vi "main_target.vi"() -> ()   [LabVIEW 2011]
uses:
  Ctrls/command.ctl
  controls.llb/RTFIFO operate.ctl
panel:
  in  "variable":T2 {"command" items=["NO_Action", "start", "pause", "resum", "stop", "config", "System_constant", "7", "DAQ_init", "DAQ_config", "DAQ_start", "DAQ_read", "DAQ_stop", "DAQ_contrl", "14", "15", "16", "17", "18", "19", "Zsf_open", "Zsf_close", "Wkf_control", "Pump_switch", "dcf_switch", "JRQ_switch"]}
  in  "error in":errorcluster
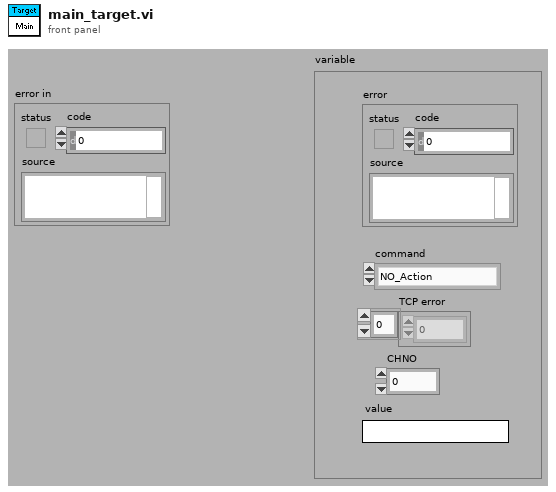
[diagram p1: front panel]
types:
  T1 = typedef "command.ctl" = u16
  T2 = cluster{"error":errorcluster, "TCP error":i32[], "command":T1, "CHNO":u16, "value":string}
  T3 = enum16{"connect", "receive data", "send data", "data transfer"}
  T4 = enum16{"connect", "receive data", "send data", "data transfer", "close"}
  T5 = typedef "RTFIFO operate.ctl" = enum16{"Creat", "Write", "Read", "Delete"}
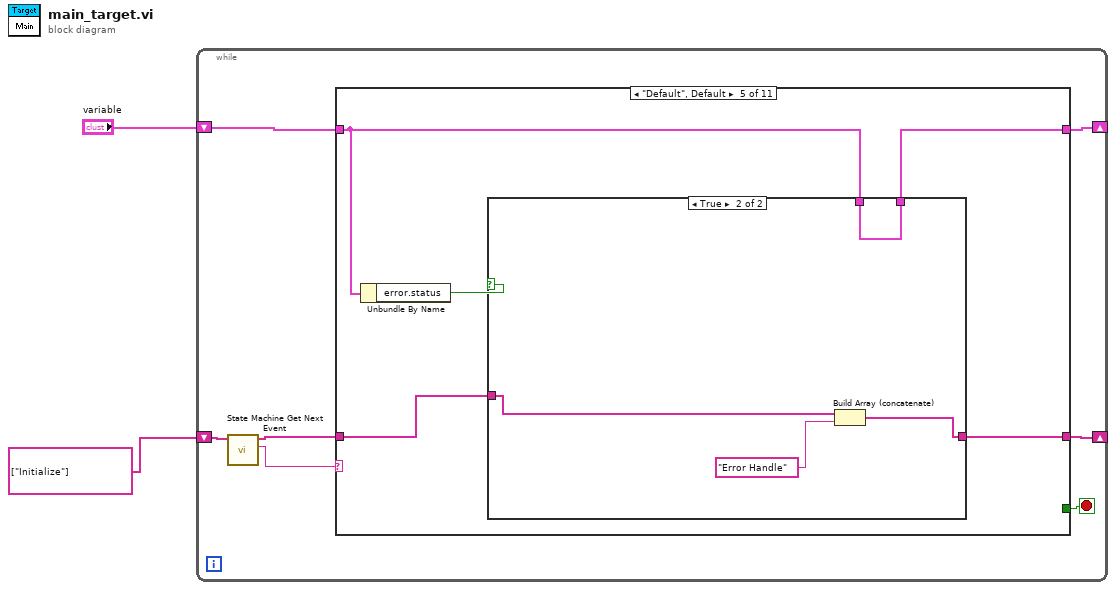
[diagram p0: block diagram]
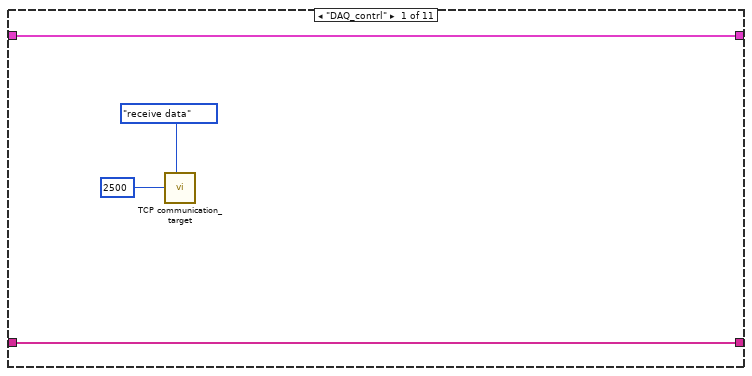
[diagram p2: hidden frame]
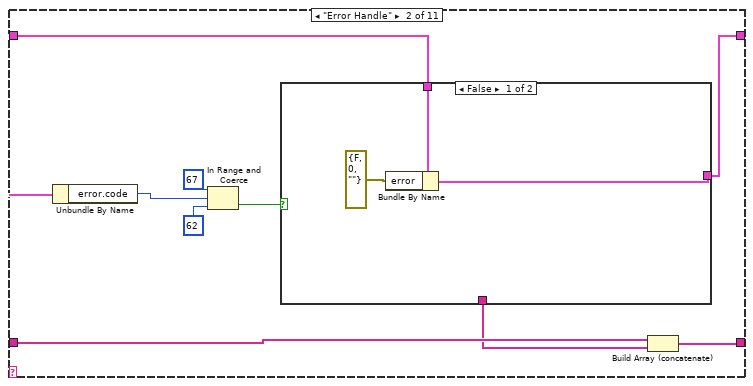
[diagram p3: hidden frame]
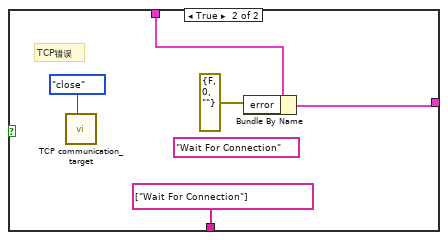
[diagram p4: hidden frame]
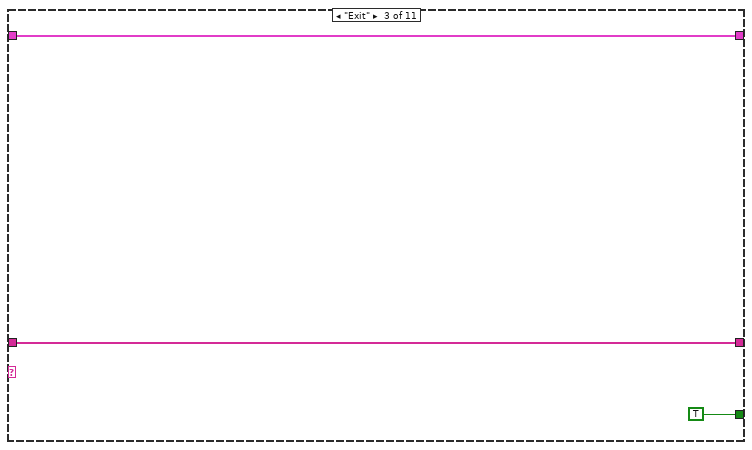
[diagram p5: hidden frame]
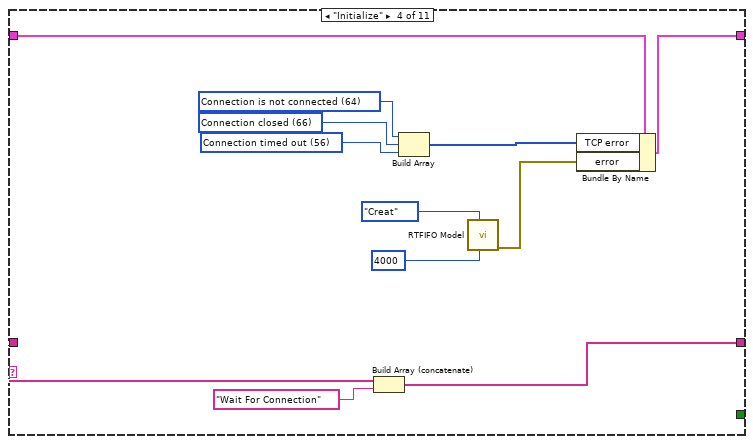
[diagram p6: hidden frame]
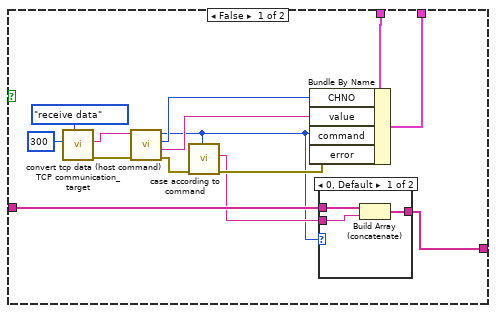
[diagram p7: hidden frame]
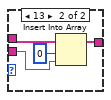
[diagram p8: hidden frame]
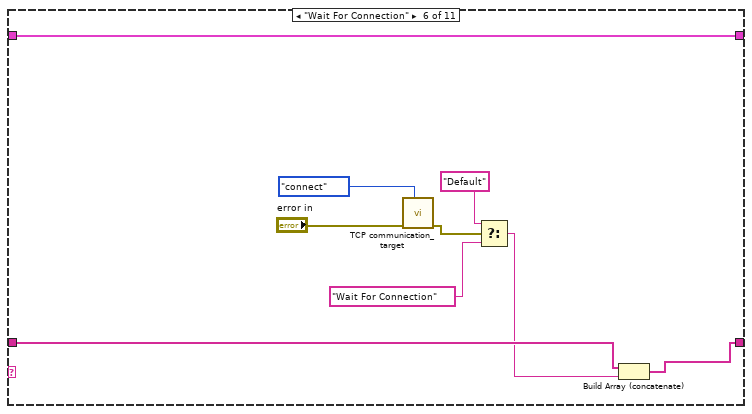
[diagram p9: hidden frame]
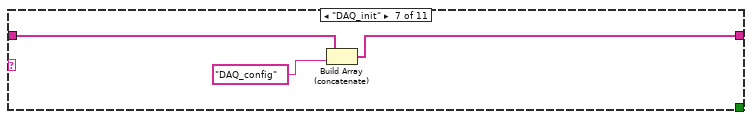
[diagram p10: hidden frame]
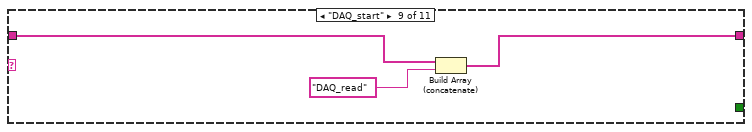
[diagram p12: hidden frame]
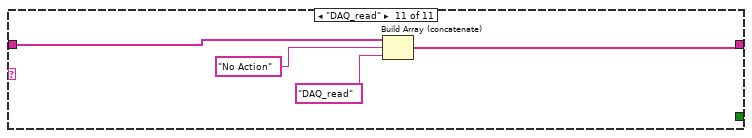
[diagram p14: hidden frame]
diagram:
  n1 = while {
    shift-right: [w5] -> _
    shift-left: string[] ["Initialize"] -> [w9]
    shift-right: [w3] -> _
    shift-left: "variable" -> [w4]
    stop <- w7 stop-if-true
    n2 = call "State Machine Get Next Event.vi"("event queue in"=w9) -> ("next event"=w8:string, "event queue out"=w6:string[])  [unwired: 5 in]
    n3 = case shown="\"Default\", Default" w8 {
      tunnel: [_ _ TRUE _ _ _ _ _ _ _ _] -> w7
      tunnel: w6 -> [w10 w20 w32 w45 w47 w78 w87 w88 w91 w93 w97]
      tunnel: [w10 w19 w32 w44 w46 w77 w86 w88 w89 w93 w96] -> w5
      tunnel: w4 -> [w13 w22 w31 w40 w50 w84 _ _ _ w92 _]
      tunnel: [w13 w21 w31 w39 w48 w84 _ _ _ w92 _] -> w3
      frame "DAQ_contrl" {
        n4 = call "TCP communication_target.vi"("TCP command"=T3."receive data", "timeout ms"=2500) -> ()  [unwired: 8 in, 2 out]
      }
      frame "Error Handle" {
        n5 = Unbundle By Name(w22) -> ("error.code"=w17:i32)
        n6 = In Range and Coerce(upper limit=67, x=w17, lower limit=62) -> (In Range?=w14:bool)  [unwired: 1 out]
        n7 = case shown="False" w14 {
          tunnel: w22 -> [w25 w29]
          tunnel: [w23 w28] -> w21
          tunnel: [_ string[] ["Wait For Connection"]] -> w18
          frame False {
            n8 = Bundle By Name(cluster=w25, "error"=errorcluster {"status"=FALSE, "code"=0, "source"=""}) -> (w23:T2)
          }
          frame True {
            (unwired) "Wait For Connection"
            # "TCP错误"
            n9 = call "TCP communication_target.vi"("TCP command"=T4."close") -> ()  [unwired: 9 in, 2 out]
            n10 = Bundle By Name(cluster=w29, "error"=errorcluster {"status"=FALSE, "code"=0, "source"=""}) -> (w28:T2)
          }
        }
        n11 = Build Array (concatenate)(w20, w18) -> (w19:string[])
      }
      frame "Exit" {
      }
      frame "Initialize" {
        w37 = 66 items=["No Error", "Argument Error", "Memory Full", "Out of Zone", "End of File", "File Already Open", "Generic File IO Error", "File Not Found", "File Permission Error", "Disk Full", "Duplicate Path", "Too Many Files Open", "Not Enabled", "Resource File Not Found", "Cannot Add Resource", "Resource Not Found", "Image Not Found", "Image Memory Error", "Pen Does Not Exist", "Config Bad Type", "Config Token Not Found", "Config Parse Error", "Config Memory Error", "Bad External Code Format", "Bad External Code Offset", "External Code Not Present", "Null Window", "Destroy Window Mixup", "Null Menu", "Print Aborted", "Bad Print Record", "Print Driver Error", "Windows Error During Print", "Memory Error During Print", "Print Dialog Error", "Generic Print Error", "Invalid Device Refnum", "Device Not Found", "Device Parameter Error", "Device Unit Error", "Can't Open Device", "Device Call Aborted", "Generic Error", "Cancelled By User", "Object ID Too Low", "Object ID Too High", "Object Not In Heap", "Unknown Heap", "Bad DefProc ID", "DefProc Not In Table", "Message Out Of Range", "Null Method", "Unknown Message", "Manager Call Not Supported", "Bad address", "Connection In progress", "Connection timed out", "Connection is already in progress", "Network attribute not supported", "Network error", "Address in use", "System out of memory", "Connection aborted", "Connection refused", "Connection is not connected", "Connection is already connected", "Connection closed", "Initialize error (interapplication manager)", "Bad occurrence", "Wait on unbound occurrence handler", "Occurrence queue overflow", "Bad path", "Semaphore not signaled", "Unrecognized type (interapplication manager)"] ("1st Error to Convert")
        w36 = 56 items=["No Error", "Argument Error", "Memory Full", "Out of Zone", "End of File", "File Already Open", "Generic File IO Error", "File Not Found", "File Permission Error", "Disk Full", "Duplicate Path", "Too Many Files Open", "Not Enabled", "Resource File Not Found", "Cannot Add Resource", "Resource Not Found", "Image Not Found", "Image Memory Error", "Pen Does Not Exist", "Config Bad Type", "Config Token Not Found", "Config Parse Error", "Config Memory Error", "Bad External Code Format", "Bad External Code Offset", "External Code Not Present", "Null Window", "Destroy Window Mixup", "Null Menu", "Print Aborted", "Bad Print Record", "Print Driver Error", "Windows Error During Print", "Memory Error During Print", "Print Dialog Error", "Generic Print Error", "Invalid Device Refnum", "Device Not Found", "Device Parameter Error", "Device Unit Error", "Can't Open Device", "Device Call Aborted", "Generic Error", "Cancelled By User", "Object ID Too Low", "Object ID Too High", "Object Not In Heap", "Unknown Heap", "Bad DefProc ID", "DefProc Not In Table", "Message Out Of Range", "Null Method", "Unknown Message", "Manager Call Not Supported", "Bad address", "Connection In progress", "Connection timed out", "Connection is already in progress", "Network attribute not supported", "Network error", "Address in use", "System out of memory", "Connection aborted", "Connection refused", "Connection is not connected", "Connection is already connected", "Connection closed", "Initialize error (interapplication manager)", "Bad occurrence", "Wait on unbound occurrence handler", "Occurrence queue overflow", "Bad path", "Semaphore not signaled", "Unrecognized type (interapplication manager)"] ("1st Error to Convert")
        w38 = 64 items=["No Error", "Argument Error", "Memory Full", "Out of Zone", "End of File", "File Already Open", "Generic File IO Error", "File Not Found", "File Permission Error", "Disk Full", "Duplicate Path", "Too Many Files Open", "Not Enabled", "Resource File Not Found", "Cannot Add Resource", "Resource Not Found", "Image Not Found", "Image Memory Error", "Pen Does Not Exist", "Config Bad Type", "Config Token Not Found", "Config Parse Error", "Config Memory Error", "Bad External Code Format", "Bad External Code Offset", "External Code Not Present", "Null Window", "Destroy Window Mixup", "Null Menu", "Print Aborted", "Bad Print Record", "Print Driver Error", "Windows Error During Print", "Memory Error During Print", "Print Dialog Error", "Generic Print Error", "Invalid Device Refnum", "Device Not Found", "Device Parameter Error", "Device Unit Error", "Can't Open Device", "Device Call Aborted", "Generic Error", "Cancelled By User", "Object ID Too Low", "Object ID Too High", "Object Not In Heap", "Unknown Heap", "Bad DefProc ID", "DefProc Not In Table", "Message Out Of Range", "Null Method", "Unknown Message", "Manager Call Not Supported", "Bad address", "Connection In progress", "Connection timed out", "Connection is already in progress", "Network attribute not supported", "Network error", "Address in use", "System out of memory", "Connection aborted", "Connection refused", "Connection is not connected", "Connection is already connected", "Connection closed", "Initialize error (interapplication manager)", "Bad occurrence", "Wait on unbound occurrence handler", "Occurrence queue overflow", "Bad path", "Semaphore not signaled", "Unrecognized type (interapplication manager)"] ("1st Error to Convert")
        n12 = Build Array (concatenate)(w45, "Wait For Connection") -> (w44:string[])
        n13 = Build Array(w38, w37, w36) -> (w35:i32[])
        n14 = call "RTFIFO Model.vi"("size"=4000, "operate"=RTFIFO_operate."Creat") -> ("error out"=w34:errorcluster)  [unwired: 8 in, 1 out]
        n15 = Bundle By Name(cluster=w40, "TCP error"=w35, "error"=w34) -> (w39:T2)
      }
      frame "Default", Default {
        n16 = Unbundle By Name(w50) -> ("error.status"=w49:bool)
        n17 = case shown="True" w49 {
          tunnel: [w61 w75] -> w48
          tunnel: w50 -> [w60 w75]
          tunnel: w47 -> [w54 w74]
          tunnel: [w51 w72] -> w46
          frame False {
            n18 = call "TCP communication_target.vi"("TCP command"=T3."receive data", "timeout ms"=300) -> ("error out"=w63:errorcluster, "data out"=w57:string)  [unwired: 8 in]
            n19 = call "convert tcp data (host command).vi"("error in"=w63, "TCP_DATA"=w57) -> ("error out"=w59:errorcluster, "value"=w55:string, "ChNo"=w56:u16, "command"=w52:T1)  [unwired: 6 in]
            n20 = call "case according to command.vi"("error in"=w59, "command"=w52) -> ("error out"=w58:errorcluster, "case"=w53:string)  [unwired: 8 in]
            n21 = Bundle By Name(cluster=w60, "CHNO"=w56, "value"=w55, "command"=w52, "error"=w58) -> (w61:T2)
            n22 = case shown="0, Default" w52 {
              tunnel: w54 -> [w67 w71]
              tunnel: [w66 w68] -> w51
              tunnel: w53 -> [w65 w70]
              frame 0, Default {
                n23 = Build Array (concatenate)(w67, w65) -> (w66:string[])
              }
              frame 13 {
                n24 = Insert Into Array(array=w71, index=0, new element=w70) -> (w68:string[])
              }
            }
          }
          frame True {
            n25 = Build Array (concatenate)(w74, "Error Handle") -> (w72:string[])
          }
        }
      }
      frame "Wait For Connection" {
        n26 = call "TCP communication_target.vi"("TCP command"=T3."connect", "error in"="error in") -> ("error out"=w81:errorcluster)  [unwired: 8 in, 1 out]
        n27 = Select(t="Default", s=w81, f="Wait For Connection") -> (s? t:f=w76:string)
        n28 = Build Array (concatenate)(w78, w76) -> (w77:string[])
      }
      frame "DAQ_init" {
        n29 = Build Array (concatenate)(w87, "DAQ_config") -> (w86:string[])
      }
      frame "DAQ_config" {
      }
      frame "DAQ_start" {
        n30 = Build Array (concatenate)(w91, "DAQ_read" ("string")) -> (w89:string[])
      }
      frame "DAQ_stop" {
      }
      frame "DAQ_read" {
        n31 = Build Array (concatenate)(w97, "No Action", "DAQ_read" ("element")) -> (w96:string[])
      }
    }
  }
